vi "forward power W subvi$.vi"(0 "VISA resource name":refnum<visa-resource-name>="GPIB0::12::INSTR", 1 "error in (no error)":errorcluster) -> (2 "VISA resource name out":refnum<visa-resource-name>, 3 "foward power (W)":dbl[unit], 4 "error out":errorcluster)   [LabVIEW 2009]
uses:
  <vilib>/regexp/Match Regular Expression.xnode
panel:
  out "read buffer":string
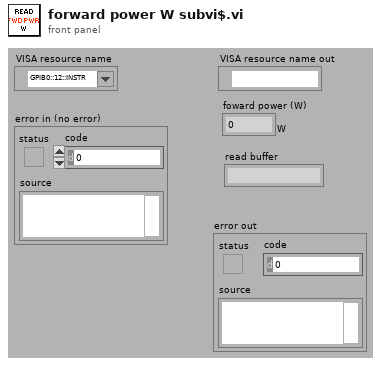
[diagram p1: front panel]
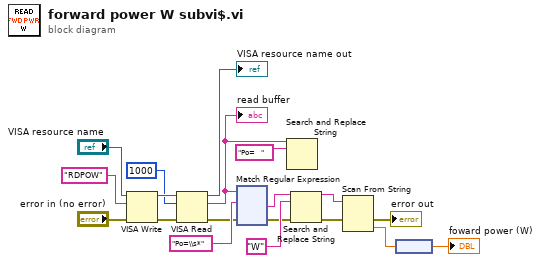
[diagram p0: block diagram]
diagram:
  n1 = VISA Write(VISA resource name="VISA resource name", write buffer="RDPOW", error in (no error)="error in (no error)") -> (VISA resource name out=w16:refnum<visa-resource-name>, error out=w17:errorcluster)  [unwired: 1 out]
  n2 = VISA Read(VISA resource name=w16, byte count=u32 1000 ("bytes to read (1000)"), error in (no error)=w17) -> (VISA resource name out=→"VISA resource name out":refnum<visa-resource-name>, read buffer=w11:string, error out=w4:errorcluster)  [unwired: 1 out]
  "read buffer" <- w11
  n3 = xnode "Match Regular Expression"("input string"=w11, "regular expression"="Po=\\s*" ("search string"), "error in"=w4) -> ("after match"=w9:string, "error out"=w3:errorcluster)  [unwired: 3 in, 3 out]
  n4 = Search and Replace String(input string=w11, search string="Po=   ") -> ()  [unwired: 6 in, 4 out]
  n5 = Search and Replace String(input string=w9, search string="W", error in=w3) -> (result string=w7:string, error out=w2:errorcluster)  [unwired: 5 in, 2 out]
  n6 = Scan From String(input string=w7, error in=w2) -> (error out=→"error out":errorcluster, output 1=w6:dbl)  [unwired: 3 in, 2 out]
  n7 = node(w6) -> (→"foward power (W)":dbl[unit])
